vi "MAIN_error_handling.vi"(3 "queue FPGA":refnum<queue>, 4 "Start acquisition":bool, 5 "queue pump":refnum<queue>, 6 "error in":errorcluster, 7 "queue valve":refnum<queue>, 8 "queue piezo":refnum<queue>, 9 "queue camera":refnum<queue>, 10 "queue ASI stage":refnum<queue>, 11 "queue DAQ":refnum<queue>) -> (0 "error out":errorcluster)   [LabVIEW 2015]
uses:
  CONTROLS/Q_DAQ_element.ctl
  CONTROLS/Q_camera_element.ctl
  CONTROLS/Q_ASI_stage_element.ctl
  CONTROLS/Q_MCL_piezo_element.ctl
  CONTROLS/Q_VALVE_element.ctl
  CONTROLS/Q_PUMP_element.ctl
  CONTROLS/Q_FPGA_element.ctl
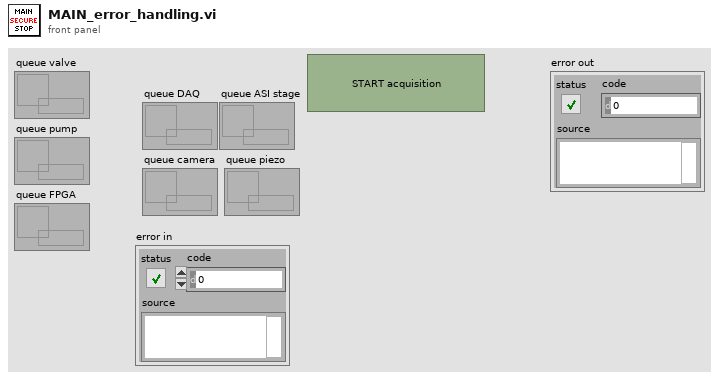
[diagram p1: front panel]
types:
  T1 = typedef "Q_FPGA_element.ctl" = cluster{"variant":variant, "Instruction":enum16{"FPGA_idle", "FPGA_initialize", "FPGA_error", "FPGA_security_stop", "FPGA_laser", "FPGA_start_stop_measure_QPD", "FPGA_measure_QPD", "FPGA_measure_QPD_noise", "FPGA_stop_measure_QPD", "FPGA_init_autofocus", "FPGA_init_single_scan", "FPGA_stop_single_scan", "FPGA_init_merFISH", "FPGA_measure_QPD_merFISH", "FPGA_init_scan_merFISH", "FPGA_scan_merFISH", "FPGA_close_merFISH", "FPGA_stop"}}
  T2 = typedef "Q_camera_element.ctl" = cluster{"variant":variant, "Instruction":enum16{"CAMERA_idle", "CAMERA_initialize", "CAMERA_error", "CAMERA_security_stop", "CAMERA_not_acquiring", "CAMERA_acquiring", "CAMERA_start_acquiring", "CAMERA_stop_acquiring", "CAMERA_change_exposure", "CAMERA_define_ROI", "CAMERA_cooler", "CAMERA_acquire_movie", "CAMERA_init_scan", "CAMERA_check_image_scan", "CAMERA_close_scan", "CAMERA_init_merFISH", "CAMERA_start_acquiring_merFISH", "CAMERA_close_scan_merFISH", "CAMERA_close_merFISH", "CAMERA_STOP"}}
  T3 = typedef "Q_PUMP_element.ctl" = cluster{"variant":variant, "Instruction":enum16{"PUMP_idle", "PUMP_initialize", "PUMP_error", "PUMP_security_stop", "PUMP_read_pressure", "PUMP_change_pressure", "PUMP_init_merFISH", "PUMP_change_presure_merFISH", "PUMP_zero_pressure_merFISH", "PUMP_close_merFISH", "PUMP_stop"}}
  T4 = typedef "Q_VALVE_element.ctl" = cluster{"variant":variant, "Instruction":enum16{"VALVE_idle", "VALVE_initialize", "VALVE_error", "VALVE_security_stop", "VALVE_change_position", "VALVE_two_way_valves", "VALVE_init_merFISH", "VALVE_stop"}}
  T5 = typedef "Q_MCL_piezo_element.ctl" = cluster{"variant":variant, "Instruction":enum16{"Piezo_idle", "Piezo_initialize", "Piezo_error", "Piezo_security_stop", "Piezo_read_z", "Piezo_move_z", "Piezo_keyboard_move", "Piezo_close_autofocus_calibration_ramp", "Piezo_change_init_state", "Piezo_init_autofocus", "Piezo_init_autofocus_merFISH_TL", "Piezo_autofocus", "Piezo_autofocus_merFISH_TL", "Piezo_stop_autofocus", "Piezo_stop_autofocus_merFISH_TL", "Piezo_autofocus_lost", "Piezo_resume_autofocus_merFISH_TL", "Piezo_check_z_position_merFISH_TL", "Piezo_init_ramp", "Piezo_move_z_ramp", "Piezo_close_ramp", "Piezo_close_merFISH", "Piezo_stop"}}
  T6 = typedef "Q_ASI_stage_element.ctl" = cluster{"variant":variant, "Instruction":enum16{"ASI_idle", "ASI_initialize", "ASI_error", "ASI_security_stop", "ASI_read_XYZ", "ASI_up", "ASI_down", "ASI_left", "ASI_right", "ASI_save_XY", "ASI_move_to_XY", "ASI_brightfield", "ASI_init_scan", "ASI_init_merFISH", "ASI_move_to_XY_merFISH", "ASI_move_to_Z_merFISH", "ASI_init_autofocus_search_merFISH", "ASI_close_autofocus_search_merFISH", "ASI_adjust_piezo_autofocus_merFISH", "ASI_set_piezo_autofocus_to_reference_position_merFISH_TL", "ASI_close_merFISH", "ASI_stop"}}
  T7 = typedef "Q_DAQ_element.ctl" = cluster{"variant":variant, "Instruction":enum16{"DAQ_idle", "DAQ_initialize", "DAQ_error", "DAQ_security_stop", "DAQ_init_single_scan", "DAQ_single_scan", "DAQ_init_merFISH", "DAQ_scan_merFISH", "DAQ_photobleaching_merFISH", "DAQ_close_merFISH", "DAQ_stop"}}
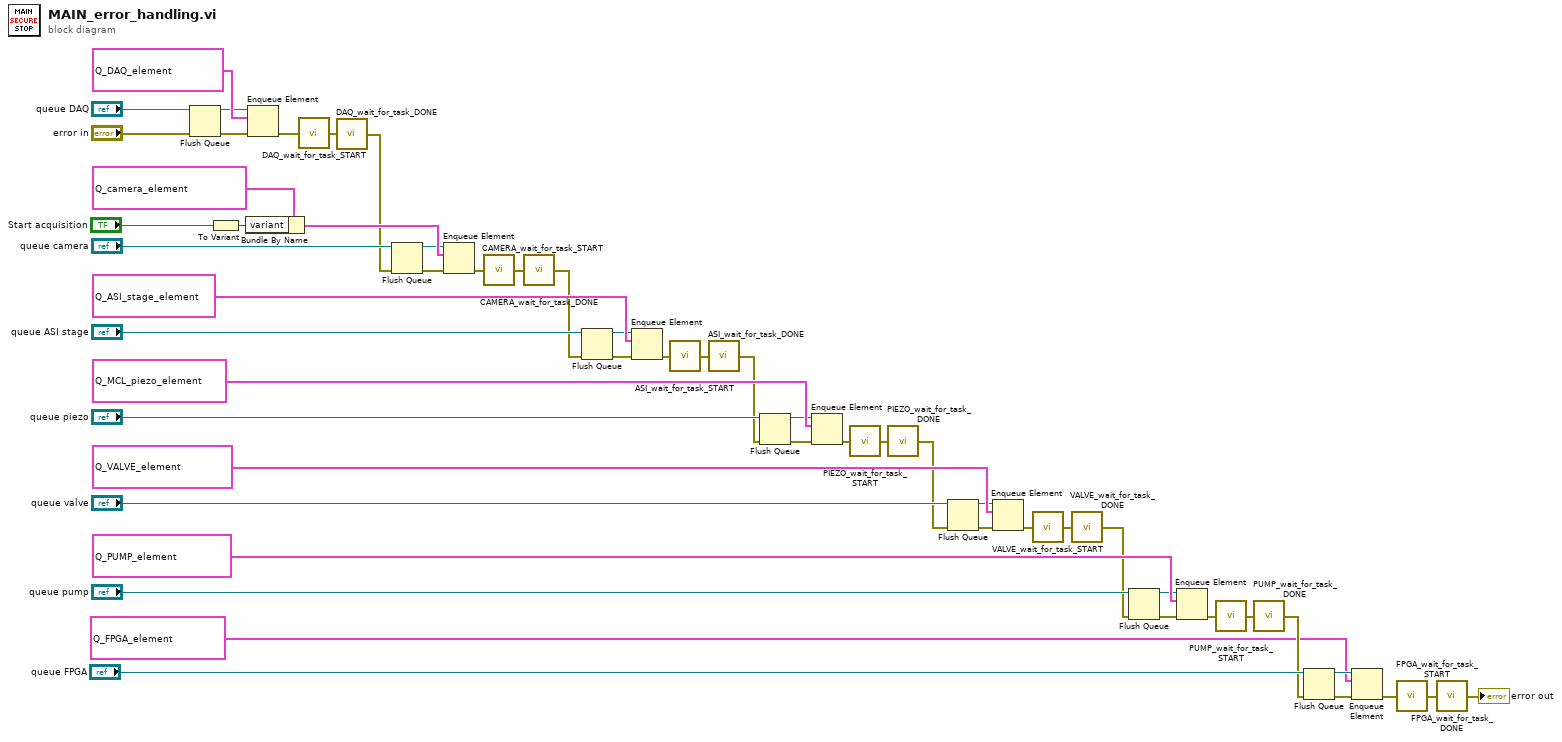
[diagram p0: block diagram]
diagram:
  n1 = Flush Queue(queue="queue DAQ", error in (no error)="error in") -> (queue out=w26:refnum<queue>, error out=w25:errorcluster)  [unwired: 1 out]
  n2 = To Variant(anything="Start acquisition") -> (Variant=w31:variant)
  n3 = Bundle By Name(cluster=T2 {"variant"=variant, "Instruction"=enum."CAMERA_security_stop"} ("Q_ANDOR_element"), "variant"=w31) -> (w32:T2)
  n4 = Enqueue Element(queue=w26, element=T7 {"variant"=variant, "Instruction"=enum."DAQ_security_stop"} ("Q_DAQ"), error in (no error)=w25) -> (error out=w1:errorcluster)  [unwired: 1 in, 2 out]
  n5 = call "DAQ_wait_for_task_START.vi"("error in"=w1) -> ("error out"=w53:errorcluster)
  n6 = call "DAQ_wait_for_task_DONE.vi"("error in"=w53) -> ("error out"=w23:errorcluster)
  n7 = Flush Queue(queue="queue camera", error in (no error)=w23) -> (queue out=w24:refnum<queue>, error out=w22:errorcluster)  [unwired: 1 out]
  n8 = Enqueue Element(queue=w24, element=w32, error in (no error)=w22) -> (error out=w34:errorcluster)  [unwired: 1 in, 2 out]
  n9 = call "CAMERA_wait_for_task_START.vi"("error in"=w34) -> ("error out"=w33:errorcluster)
  n10 = call "CAMERA_wait_for_task_DONE.vi"("error in"=w33) -> ("error out"=w20:errorcluster)
  n11 = Flush Queue(queue="queue ASI stage", error in (no error)=w20) -> (queue out=w21:refnum<queue>, error out=w19:errorcluster)  [unwired: 1 out]
  n12 = Enqueue Element(queue=w21, element=T6 {"variant"=variant, "Instruction"=enum."ASI_security_stop"} ("Q_ASI_stage"), error in (no error)=w19) -> (error out=w49:errorcluster)  [unwired: 1 in, 2 out]
  n13 = call "ASI_wait_for_task_START.vi"("error in"=w49) -> ("error out"=w48:errorcluster)
  n14 = call "ASI_wait_for_task_DONE.vi"("error in"=w48) -> ("error out"=w16:errorcluster)
  n15 = Flush Queue(queue="queue piezo", error in (no error)=w16) -> (queue out=w18:refnum<queue>, error out=w17:errorcluster)  [unwired: 1 out]
  n16 = Enqueue Element(queue=w18, element=T5 {"variant"=variant, "Instruction"=enum."Piezo_security_stop"} ("Q_MCL_Piezo"), error in (no error)=w17) -> (error out=w45:errorcluster)  [unwired: 1 in, 2 out]
  n17 = call "PIEZO_wait_for_task_START.vi"("error in"=w45) -> ("error out"=w44:errorcluster)
  n18 = call "PIEZO_wait_for_task_DONE.vi"("error in"=w44) -> ("error out"=w14:errorcluster)
  n19 = Flush Queue(queue="queue valve", error in (no error)=w14) -> (queue out=w15:refnum<queue>, error out=w11:errorcluster)  [unwired: 1 out]
  n20 = Enqueue Element(queue=w15, element=T4 {"variant"=variant, "Instruction"=enum."VALVE_security_stop"}, error in (no error)=w11) -> (error out=w42:errorcluster)  [unwired: 1 in, 2 out]
  n21 = call "VALVE_wait_for_task_START.vi"("error in"=w42) -> ("error out"=w43:errorcluster)
  n22 = call "VALVE_wait_for_task_DONE.vi"("error in"=w43) -> ("error out"=w12:errorcluster)
  n23 = Flush Queue(queue="queue pump", error in (no error)=w12) -> (queue out=w13:refnum<queue>, error out=w10:errorcluster)  [unwired: 1 out]
  n24 = Enqueue Element(queue=w13, element=T3 {"variant"=variant, "Instruction"=enum."PUMP_security_stop"}, error in (no error)=w10) -> (error out=w39:errorcluster)  [unwired: 1 in, 2 out]
  n25 = call "PUMP_wait_for_task_START.vi"("error in"=w39) -> ("error out"=w38:errorcluster)
  n26 = call "PUMP_wait_for_task_DONE.vi"("error in"=w38) -> ("error out"=w7:errorcluster)
  n27 = Flush Queue(queue="queue FPGA", error in (no error)=w7) -> (queue out=w6:refnum<queue>, error out=w9:errorcluster)  [unwired: 1 out]
  n28 = Enqueue Element(queue=w6, element=T1 {"variant"=variant, "Instruction"=enum."FPGA_security_stop"}, error in (no error)=w9) -> (error out=w4:errorcluster)  [unwired: 1 in, 2 out]
  n29 = call "FPGA_wait_for_task_START.vi"("error in"=w4) -> ("error out"=w3:errorcluster)
  n30 = call "FPGA_wait_for_task_DONE.vi"("error in"=w3) -> ("error out"=→"error out":errorcluster)
